vi "_txtData Spectrum.vi"(5 "Spectrum":i32[](array[numeric]), 7 "id":i32=1) -> (3 "Output Text":string)   [LabVIEW 2012]
uses:
  Configuration/_Global Configuration.vi
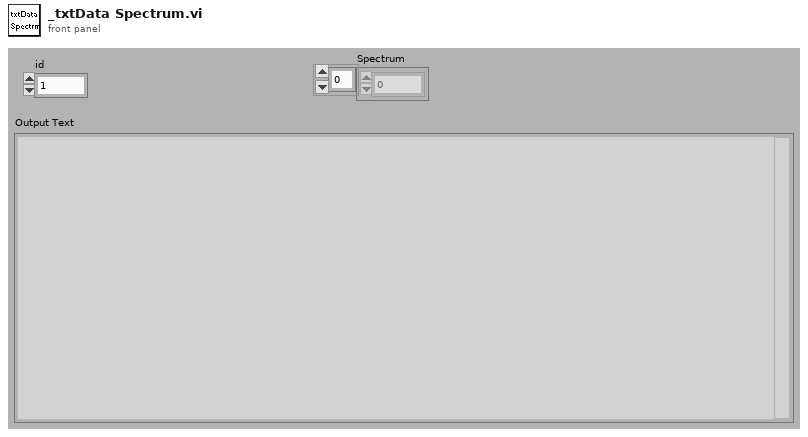
[diagram p1: front panel]
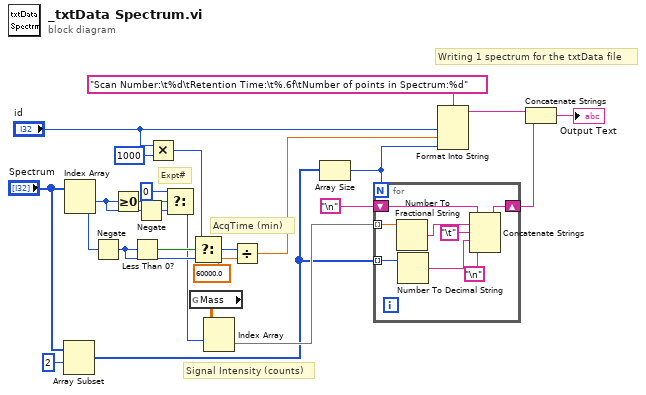
[diagram p0: block diagram]
diagram:
  # "Signal Intensity (counts)"
  # "AcqTime (min)"
  # "Expt#"
  # "Writing 1 spectrum for the txtData file"
  n1 = Array Subset(array="Spectrum", index=2) -> (w3:i32[])  [unwired: 1 in]
  n2 = Index Array(array="Spectrum") -> (element #1=w22:i32, element #2=w19:i32)  [unwired: 2 in]
  n3 = Negate(x=w19) -> (-x=w17:i32)
  n4 = Greater Or Equal To 0?(x=w22) -> (x >= 0?=w23:bool)
  n5 = Less Than 0?(x=w17) -> (x < 0?=w18:bool)
  n6 = Negate(x=w22) -> (-x=w21:i32)
  n7 = Multiply(x="id", y=1000) -> (x*y=w15:i32)
  n8 = Select(t=0, s=w23, f=w21) -> (s? t:f=w9:i32)
  n9 = global read "_Global Configuration.vi" "Mass"() -> (w10:dbl[][])
  n10 = Select(t=w15, s=w18, f=w17) -> (s? t:f=w14:i32)
  n11 = Index Array(array=w10, index (row)=w9) -> (element=w4:dbl[])  [unwired: 1 in]
  n12 = Divide(x=w14, y=60000.0) -> (x/y=w7:dbl)
  n13 = Array Size(array=w3) -> (size(s)=w5:i32)
  n14 = for {
    N: w5 -> [_]
    tunnel: w4 -> [w33] mode=indexing
    shift-right: [w30] -> w1
    shift-left: "\n" -> [w31]
    tunnel: w3 -> [w29] mode=indexing
    n15 = Number To Fractional String(number=w33) -> (F-format string=w32:string)  [unwired: 3 out]
    n16 = Number To Decimal String(number=w29) -> (decimal integer string=w28:string)  [unwired: 1 out]
    n17 = Concatenate Strings(w31, w32, "\t", w28, "\n") -> (w30:string)
  }
  n18 = Format Into String(format string="Scan Number:\t%d\tRetention Time:\t%.6f\tNumber of points in Spectrum:%d", "id", w7, w5) -> (resulting string=w2:string)  [unwired: 2 in, 1 out]
  n19 = Concatenate Strings(w2, w1) -> (→"Output Text":string)
